vi "Set Bias Voltage.vi"(8 "error in (no error)":errorcluster, 9 "Channel":i32, 10 "Bias Voltage (V)":dbl, 11 "Example in":refnum<class "Instrument.Template.lvclass">) -> (0 "error out":errorcluster, 3 "Example out":refnum<class "Instrument.Template.lvclass">)   [LabVIEW 2019, in "Instrument.Template.lvclass"]
uses:
  Instrument.Template.lvclass
  C:/Users/patrick/Documents/GitHub/Instrument-Framework/lvsrc/SMOs/Instrument/Instrument.lvclass
  Typedefs/Instrument.Template.Commands--Enum.ctl
  SMOs/Instrument/Instrument.lvclass/Instrument.ctl
  67792bfe-8e2c-4879-abc2-cb448bcec168.vi
  67792bfe-8e2c-4879-abc2-cb448bcec168.vi/d2bb5a9c-a26b-4ca4-a4cc-5416167f039a.vi
  SMOs/Instrument/API/Send and Receive.vi
  67792bfe-8e2c-4879-abc2-cb448bcec168.vi/5bdfcc90-4ab6-4bd0-b0c8-d29eb6fbf966.vi
  SMOs/Instrument/Private/Get Client Type.vi
  67792bfe-8e2c-4879-abc2-cb448bcec168.vi/d2bb5a9c-a26b-4ca4-a4cc-5416167f039a.vi/82809fde-cc3a-40f5-b2ef-425d34fbb2ab.vi
  67792bfe-8e2c-4879-abc2-cb448bcec168.vi/d2bb5a9c-a26b-4ca4-a4cc-5416167f039a.vi/f30b6d1c-8129-4f04-876b-dc9c63ddac9f.vi
  67792bfe-8e2c-4879-abc2-cb448bcec168.vi/5bdfcc90-4ab6-4bd0-b0c8-d29eb6fbf966.vi/c71b15aa-0cc9-4698-a5bb-aec5a86ae631.vi
  67792bfe-8e2c-4879-abc2-cb448bcec168.vi/5bdfcc90-4ab6-4bd0-b0c8-d29eb6fbf966.vi/c71b15aa-0cc9-4698-a5bb-aec5a86ae631.vi/6221cf9c-6d86-4c77-aafd-cc8725942eea.vi
  67792bfe-8e2c-4879-abc2-cb448bcec168.vi/5bdfcc90-4ab6-4bd0-b0c8-d29eb6fbf966.vi/c71b15aa-0cc9-4698-a5bb-aec5a86ae631.vi/cc0d689a-903c-4928-8477-97c8b01fef90.vi
  SMOs/Instrument/Private/Get RC Connection Status.vi
  SMOs/Instrument/API/Enum to String.vi
  SMOs/RemoteControl/API/Send and Receive.vi
  <vilib>/Utility/Data Type/Get Type Information.vi
  <vilib>/JDP Science/JSONtext/JSON text to Variant.vi
  <vilib>/National Instruments/GUID Generator/Guid Generator.vi
  SMOs/Instrument/API/Instrument.GetPublicEvents.vi
  SMOs/Instrument/API/Instrument.MessageToProcess.vi
  SMOs/Instrument/Private/Instrument.MessageFromProcess.EventStructure.vi
  <vilib>/JDP Science/JSONtext/LVClass Serializer/JSONtext LVClass Serializer.lvclass
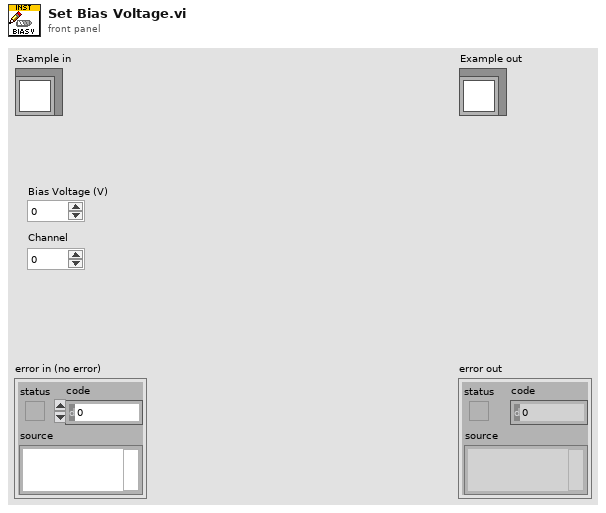
[diagram p1: front panel]
types:
  T1 = typedef "Instrument.Template.lvclass/Instrument.Template.Commands--Enum.ctl" = enum16{"command0", "command1", "command2"}
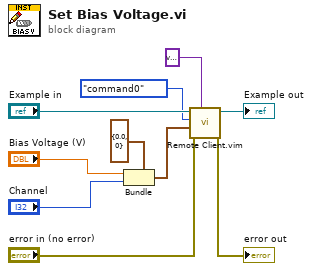
[diagram p0: block diagram]
diagram:
  n1 = Bundle(cluster=cluster{"Bias Voltage (V)":dbl, "Channel":i32} {"Bias Voltage (V)"=0.0, "Channel"=0} ("output cluster"), "Bias Voltage (V)"="Bias Voltage (V)", "Channel"="Channel") -> (w3:cluster{"Bias Voltage (V)":dbl, "Channel":i32})
  n2 = call "Remote Client.vim"("Data Out type"=variant, "error in (no error)"="error in (no error)", "params"=w3, "method"=Instrument.Template.Commands--Enum."command0" ("Commands"), "Instrument in"="Example in") -> ("error out"=→"error out":errorcluster, "Instrument out"=→"Example out":refnum<class "Instrument.Template.lvclass">)  [unwired: 3 in, 2 out]
